vi "Select Mode Dialog.vi"(8 "error in":errorcluster, 10 "Comp/Check in":T1) -> (0 "error out":errorcluster, 2 "Comp/Check out":T1, 3 "OK?":bool)   [LabVIEW 2020, in "GUCalibration2.lvlib"]
uses:
  GUCalibration2.lvlib
  Controls/CalibrationOrCheck.ctl
panel:
  in  "Abort":bool
  in  "Cal or Check":T1
  in  "OK":bool
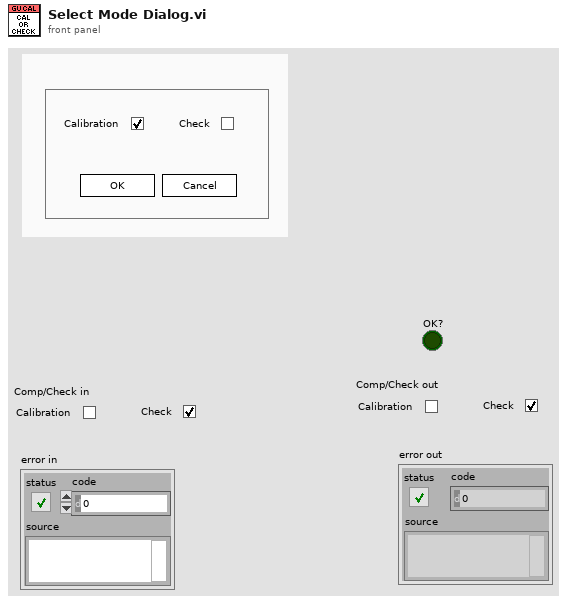
[diagram p1: front panel]
types:
  T1 = typedef "GUCalibration2.lvlib/CalibrationOrCheck.ctl" = enum32{"Calibration", "Check"}
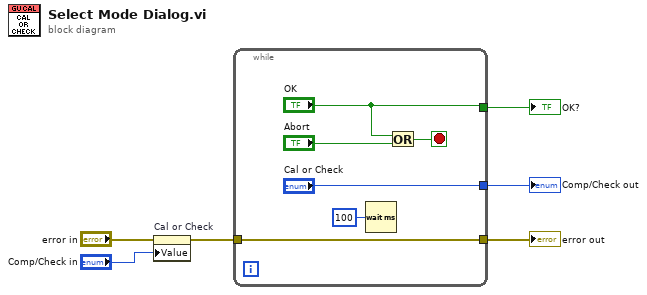
[diagram p0: block diagram]
diagram:
  n1 = property on="Cal or Check" class="RadioBtnsControl (strict)"(error in="error in", "Value"="Comp/Check in") -> (error out=w2:errorcluster)  [unwired: 1 in, 1 out]
  n2 = while {
    tunnel: ["OK"] -> w6
    tunnel: ["Cal or Check"] -> w4
    tunnel: w2 -> [w11]
    tunnel: [w11] -> w5
    stop <- w7 stop-if-true
    n3 = Wait (ms)(milliseconds to wait=u32 100) -> ()  [unwired: 1 out]
    n4 = Or(x="OK", y="Abort") -> (x .or. y?=w7:bool)
  }
  "OK?" <- w6
  "error out" <- w5
  "Comp/Check out" <- w4
